vi "General Configuration.vi"(11 "Controller In":refnum<class "gController.lvclass">) -> ()   [LabVIEW 2016, in "Controller.lvlib"]
uses:
  Controller.lvlib
  <vilib>/Utility/config.llb/NI_LVConfig.lvlib
  <vilib>/Utility/config.llb/Read Key (U32).vi
  Messages/Change Filter MSG/Change Filter Position MSG.lvclass
  <vilib>/ActorFramework/Message Enqueuer/Message Enqueuer.lvclass
  <vilib>/Utility/config.llb/Read Key (Boolean).vi
  Messages/Update Vacuum Pump State MSG/Update Vacuum Pump State MSG.lvclass
  Messages/Enable Fan MSG/Enable Fan MSG.lvclass
  <vilib>/Utility/config.llb/Read Key (Double).vi
  Messages/Update Fan Voltage MSG/Update Fan Voltage MSG.lvclass
  Messages/Toggle USB MSG/Toggle USB MSG.lvclass
  Messages/Toggle AC Spare MSG/Toggle AC Spare MSG.lvclass
  Messages/Save Data MSG/Save Data MSG.lvclass
  <vilib>/ActorFramework/Actor/Actor.lvclass
  gController.lvclass
  C:/Program Files (x86)/National Instruments/LabVIEW 2016/vi.lib/MSR Consulting, LLC/General Reuse/SuperActor/SuperActor.lvclass
  C:/Program Files (x86)/National Instruments/LabVIEW 2016/vi.lib/ActorFramework/Actor/Actor.lvclass
  C:/Program Files (x86)/National Instruments/LabVIEW 2016/vi.lib/ActorFramework/Message/Message.lvclass
  G:/sw_repo/For Builds/Nicholas/Controller/Messages/Generic Boolean MSG/Generic Boolean Message.lvclass
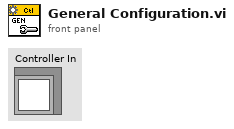
[diagram p1: front panel]
types:
  T1 = typedef "NI_LVConfig.lvlib/Config Data RefNum.ctl" = refnum<k1>
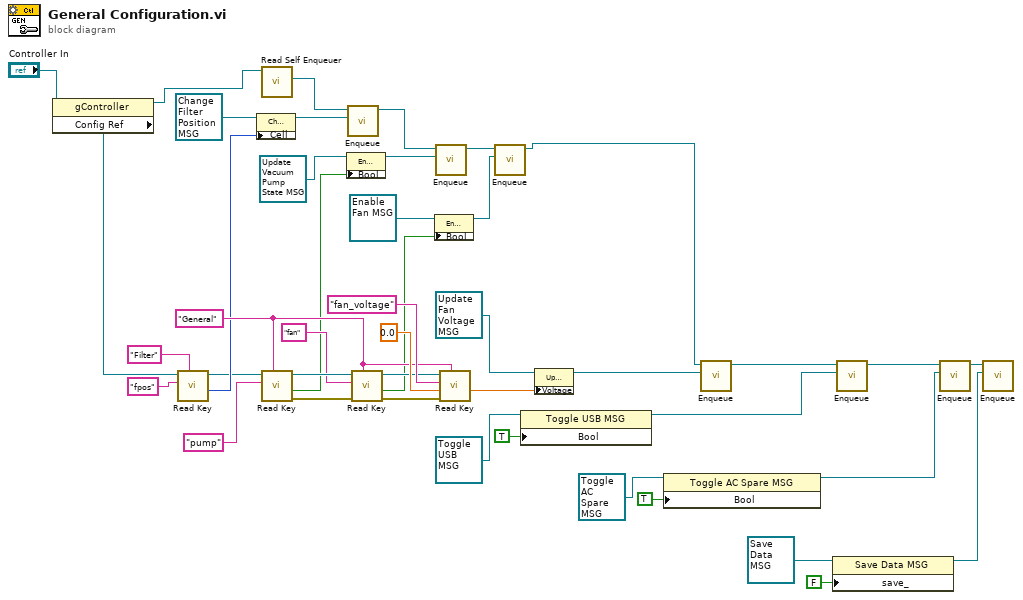
[diagram p0: block diagram]
diagram:
  w23 = "General" ("section")
  n1 = property class="gController"(reference="Controller In") -> (reference out=w2:refnum<class "gController.lvclass">, "Config Ref"=w3:T1)  [unwired: 1 in, 1 out]
  n2 = call-poly <vilib>:"Read Key.vi"("section"="Filter", "key"="fpos", "refnum"=w3) -> ("value"=w8:u32, "refnum out"=w6:T1)  [unwired: 5 in, 2 out]
  n3 = property class="Change Filter Position"(reference=refnum<class "Change Filter Position MSG.lvclass"> refnum ("Controller.lvlib:Change Filter Position"), "Cell"=w8) -> (reference out=w9:refnum<class "Change Filter Position MSG.lvclass">)  [unwired: 1 in, 1 out]
  n4 = call <vilib>:"Read Self Enqueuer.vi"("Actor"=w2) -> ("Self Enqueuer"=w42:refnum<class "Message Enqueuer.lvclass">)  [unwired: 10 in]
  n5 = call-poly <vilib>:"Read Key.vi"("section"=w23, "key"="pump", "refnum"=w6) -> ("error out"=w16:errorcluster, "value"=w14:bool, "refnum out"=w18:T1)  [unwired: 5 in, 1 out]
  n6 = property class="Enable Vacuum Pump MSG"(reference=refnum<class "Update Vacuum Pump State MSG.lvclass"> refnum ("Controller.lvlib:Enable Vacuum Pump MSG"), "Bool"=w14) -> (reference out=w15:refnum<class "Update Vacuum Pump State MSG.lvclass">)  [unwired: 1 in, 1 out]
  n7 = call <vilib>:"Enqueue.vi"("Message"=w9, "Message Enqueuer in"=w42) -> ("Message Enqueuer out"=w12:refnum<class "Message Enqueuer.lvclass">)  [unwired: 8 in, 1 out]
  n8 = call-poly <vilib>:"Read Key.vi"("section"=w23, "error in (no error)"=w16, "key"="fan", "refnum"=w18) -> ("error out"=w25:errorcluster, "value"=w20:bool, "refnum out"=w22:T1)  [unwired: 4 in, 1 out]
  n9 = property class="Enable Compressor MSG"(reference=refnum<class "Enable Fan MSG.lvclass"> refnum ("Controller.lvlib:Enable Compressor MSG"), "Bool"=w20) -> (reference out=w21:refnum<class "Enable Fan MSG.lvclass">)  [unwired: 1 in, 1 out]
  n10 = call <vilib>:"Enqueue.vi"("Message"=w15, "Message Enqueuer in"=w12) -> ("Message Enqueuer out"=w43:refnum<class "Message Enqueuer.lvclass">)  [unwired: 8 in, 1 out]
  n11 = call-poly <vilib>:"Read Key.vi"("section"=w23, "error in (no error)"=w25, "default value"=0.0, "key"="fan_voltage", "refnum"=w22) -> ("value"=w28:dbl)  [unwired: 3 in, 3 out]
  n12 = call <vilib>:"Enqueue.vi"("Message"=w21, "Message Enqueuer in"=w43) -> ("Message Enqueuer out"=w1:refnum<class "Message Enqueuer.lvclass">)  [unwired: 8 in, 1 out]
  n13 = property class="Toggle USB MSG"(reference=refnum<class "Toggle USB MSG.lvclass"> refnum ("Controller.lvlib:Toggle USB MSG"), "Bool"=TRUE) -> (reference out=w32:refnum<class "Toggle USB MSG.lvclass">)  [unwired: 1 in, 1 out]
  n14 = property class="Update Fan Voltage MSG"(reference=refnum<class "Update Fan Voltage MSG.lvclass"> refnum ("Controller.lvlib:Update Fan Voltage MSG"), "Voltage"=w28) -> (reference out=w29:refnum<class "Update Fan Voltage MSG.lvclass">)  [unwired: 1 in, 1 out]
  n15 = property class="Toggle AC Spare MSG"(reference=refnum<class "Toggle AC Spare MSG.lvclass"> refnum ("Controller.lvlib:Toggle AC Spare MSG"), "Bool"=TRUE) -> (reference out=w37:refnum<class "Toggle AC Spare MSG.lvclass">)  [unwired: 1 in, 1 out]
  n16 = call <vilib>:"Enqueue.vi"("Message"=w29, "Message Enqueuer in"=w1) -> ("Message Enqueuer out"=w33:refnum<class "Message Enqueuer.lvclass">)  [unwired: 8 in, 1 out]
  n17 = property class="Save Data MSG"(reference=refnum<class "Save Data MSG.lvclass"> refnum ("Controller.lvlib:Save Data MSG"), "save_"=FALSE) -> (reference out=w41:refnum<class "Save Data MSG.lvclass">)  [unwired: 1 in, 1 out]
  n18 = call <vilib>:"Enqueue.vi"("Message"=w32, "Message Enqueuer in"=w33) -> ("Message Enqueuer out"=w34:refnum<class "Message Enqueuer.lvclass">)  [unwired: 8 in, 1 out]
  n19 = call <vilib>:"Enqueue.vi"("Message"=w37, "Message Enqueuer in"=w34) -> ("Message Enqueuer out"=w38:refnum<class "Message Enqueuer.lvclass">)  [unwired: 8 in, 1 out]
  n20 = call <vilib>:"Enqueue.vi"("Message"=w41, "Message Enqueuer in"=w38) -> ()  [unwired: 8 in, 2 out]
